vi "Midbrain.vi"() -> ()   [LabVIEW 2010]
doc: "This VI acts as the MIDbrain in the Olin Robotics Architecture. It interacts with neural clusters on both the Forebrain and Hindbrain as shown in teh respective control panel dynamic documentation diagrams."
uses:
  <vilib>/Platform/TimedLoop/XDataNode/XDataNode.xnode
  <vilib>/Platform/TimedLoop/XDataNode/timing_clust.ctl
  <vilib>/Platform/TimedLoop/XDataNode/nitl_modes.ctl
  <vilib>/Platform/TimedLoop/XDataNode/wakeup.ctl
  GlobalHowAmI.vi
  GlobalACT.vi
  GlobalWhatAroundMe.vi
  GlobalWhereAmI.vi
  <vilib>/Platform/TimedLoop/XDataNode/XDNodeRunTimeDep.lvlib
panel:
  out "Lane Follow":dbl[](array[numeric])
  out "Wall Follow":dbl[](array[numeric])
  out "AvoidWall":dbl[](array[numeric])
  out "ObsAvoid":dbl[](array[numeric])
  out "ActCommand":dbl[](array[numeric])
  out "Act Command":cluster{"Velocity":dbl, "Direction":dbl}
  out "WhereAmI? Clean":T1
  out "HowAmI? Clean":cluster{"T":dbl, "Battery":dbl, "Temp":dbl}
  out "WhatAroundMe? Clean":cluster{"T":dbl, "Range":dbl, "Bearing":dbl}[](array[cluster])
  out "Cerr":bool
  out "Limbic":bool
  out "How?":bool
  out "Act":bool
  out "What?":bool
  in  "RT-stop":bool
  out "Where?":bool
  # "must un-stop for new run"
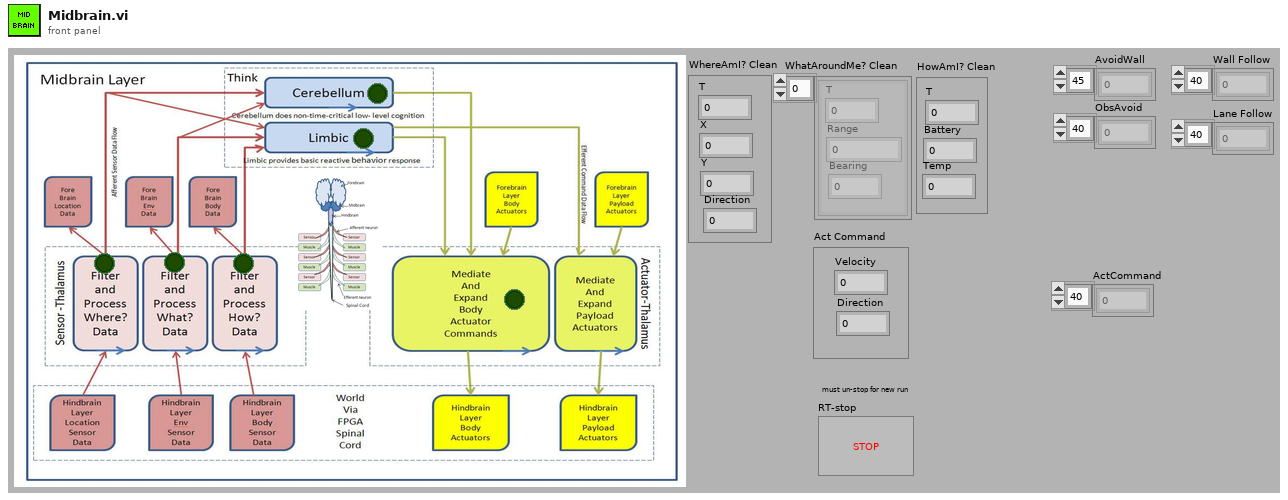
[diagram p1: front panel]
types:
  T1 = cluster{"T":dbl, "X":dbl, "Y":dbl, "Direction":dbl}
  T2 = typedef "XDNodeRunTimeDep.lvlib/timing_clust.ctl" = cluster{"Expected End [f-1]":u64, "Actual End [f-1]":u64, "Finished Late? [f-1]":bool, "Expected End [i-1]":u64, "Actual End [i-1]":u64, "Finished Late? [i-1]":bool, "Expected Start [i]":u64, "Actual Start [i]":u64, "Expected Start [f]":u64, "Actual Start [f]":u64, "Source Name":string, "Structure Name":string, "Period":i64, "Deadline":i64, "Offset":i64, "Start":i64, "Priority":i32, "Timeout":i32, "Mode":T3, "Wakeup Reason":T4, "Error":errorcluster, "Source Type":string, "Secondary Source Type":string, "Global End Time":u64, "Global Start Time":u64, "Frame Duration":u64, "Iteration Duration":u64, "Assigned CPU":i32, "I/O Scan Engine Mode":u32}
  T3 = typedef "XDNodeRunTimeDep.lvlib/nitl_modes.ctl" = enum32{"No Change", "Process missed periods, maintain original phase", "Discard missed periods, maintain original phase", "Process missed periods, ignore original phase", "Discard missed periods, ignore original phase"}
  T4 = typedef "XDNodeRunTimeDep.lvlib/wakeup.ctl" = enum32{"Normal", "Aborted", "Asynchronous wakeup", "Timing source error", "Timed loop error", "Timeout"}
  T5 = cluster{"VelCom":dbl, "BehCom":enum16{"OpenFieldTransit", "WallFollow", "LaneFollow", "ManualMode"}}
  T6 = cluster{"AvoidWall":bool, "Wander":bool, "WallFollow":bool, "LaneFollow":bool}
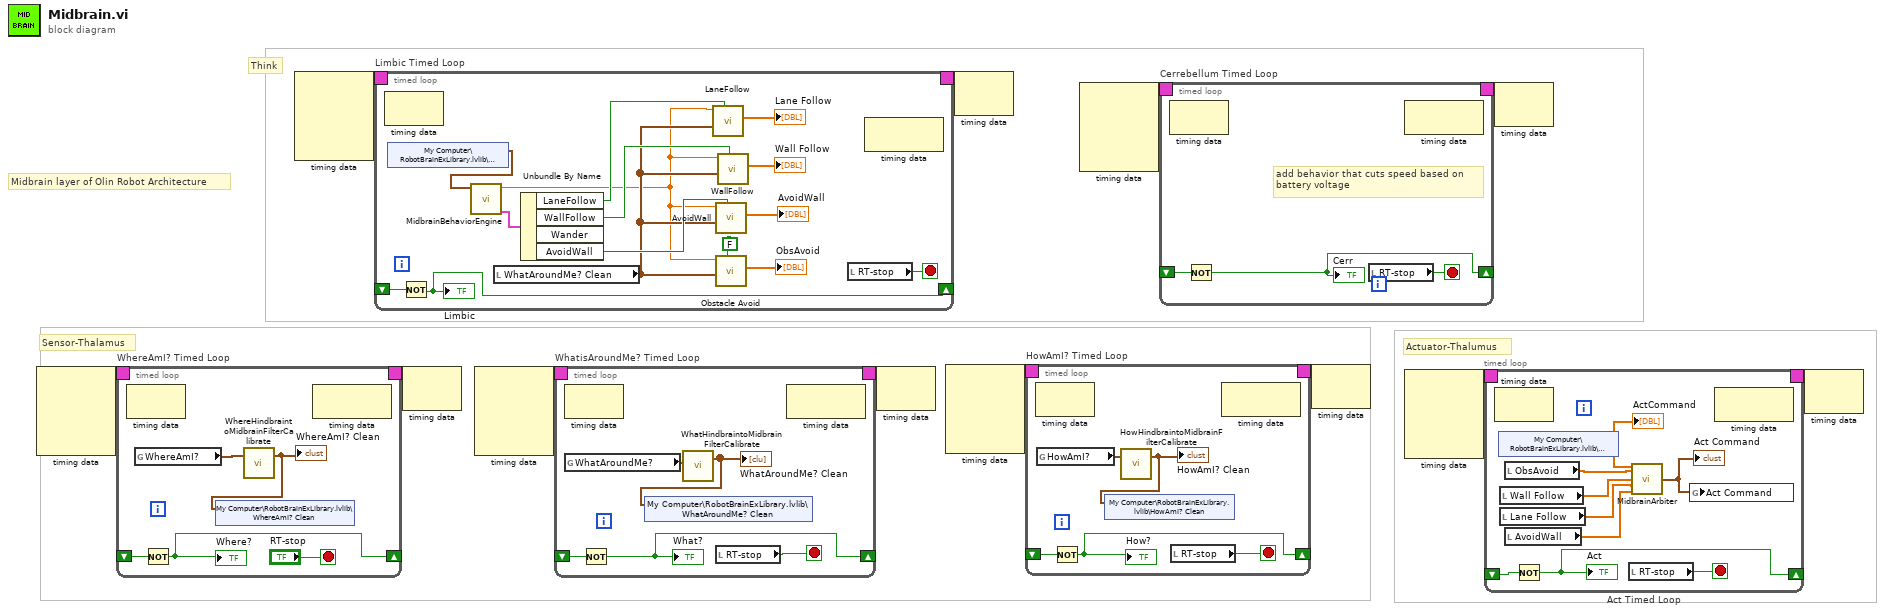
[diagram p0: block diagram]
diagram:
  # "Midbrain layer of Olin Robot Architecture"
  # "Think"
  # "Actuator-Thalumus"
  # "Sensor-Thalamus"
  n1 = node-c288 ("Input Node")() -> (w12:T2)  [unwired: 4 in]
  n2 = timed-loop "WhereAmI? Timed Loop" {
    timing: w12 -> [_]
    timing-out: [_] -> w11
    shift-right: [w16] -> _
    shift-left: _ -> [w17]
    stop <- "RT-stop" stop-if-true
    n3 = node-c288() -> ()  [unwired: 1 in, 1 out]
    n4 = global read "GlobalWhereAmI.vi" "WhereAmI?"() -> (w14:T1)
    n5 = Not(x=w17) -> (.not. x?=w16:bool)
    "Where?" <- w16
    n6 = call "WhereHindbraintoMidbrainFilterCalibrate.vi"("WhereAmI? Raw"=w14) -> ("WhereAmI? Clean"=w13:T1)  [unwired: 2 in]
    "WhereAmI? Clean" <- w13
    n7 = shared-variable "My Computer\\RobotBrainExLibrary.lvlib\\WhereAmI? Clean"(w13) -> ()  [unwired: 1 in, 1 out]
    n8 = node-c288() -> ()  [unwired: 1 in, 1 out]
  }
  n9 = node-c288 ("Input Node")() -> (w4:T2)  [unwired: 4 in]
  n10 = timed-loop "Limbic Timed Loop" {
    timing: w4 -> [_]
    timing-out: [_] -> w3
    shift-right: [w27] -> _
    shift-left: _ -> [w34]
    stop <- w33 stop-if-true
    n11 = node-c288() -> ()  [unwired: 1 in, 1 out]
    n12 = shared-variable "My Computer\\RobotBrainExLibrary.lvlib\\ForebrainCom"() -> (w31:T5)  [unwired: 1 in, 1 out]
    n13 = Not(x=w34) -> (.not. x?=w27:bool)
    "Limbic" <- w27
    n14 = call "MidbrainBehaviorEngine.vi"("ForebrainCom"=w31) -> ("BehaviorInhibit"=w26:T6, "VelCom"=w21:dbl)  [unwired: 9 in]
    n15 = local read "WhatAroundMe? Clean"() -> (w23:cluster{"T":dbl, "Range":dbl, "Bearing":dbl}[])
    n16 = Unbundle By Name(w26) -> ("LaneFollow"=w22:bool, "WallFollow"=w24:bool, "AvoidWall"=w25:bool)  [unwired: 1 out]
    n17 = call "LaneFollow.vi"("Inhibit"=w22, "WhatAroundMe? Clean"=w23, "Velocity"=w21) -> ("ActCommand"=→"Lane Follow":dbl[])  [unwired: 6 in, 2 out]
    n18 = call "AvoidWall.vi"("Inhibit"=w25, "WhatAroundMe? Clean"=w23, "Velocity"=w21) -> ("ActCommand"=→"AvoidWall":dbl[])  [unwired: 7 in, 1 out]
    n19 = call "Obstacle Avoid.vi"("Inhibit"=FALSE, "WhatAroundMe? Clean"=w23, "VelCom"=w21) -> ("ActCommand"=→"ObsAvoid":dbl[])  [unwired: 7 in, 1 out]
    n20 = call "WallFollow.vi"("Inhibit"=w24, "WhatAroundMe? Clean"=w23, "Velocity"=w21) -> ("ActCommand"=→"Wall Follow":dbl[])  [unwired: 6 in, 2 out]
    n21 = local read "RT-stop"() -> (w33:bool)
    n22 = node-c288() -> ()  [unwired: 1 in, 1 out]
  }
  n23 = node-c288(w11) -> ()  [unwired: 1 out]
  n24 = node-c288 ("Input Node")() -> (w10:T2)  [unwired: 4 in]
  n25 = timed-loop "WhatisAroundMe? Timed Loop" {
    timing: w10 -> [_]
    timing-out: [_] -> w9
    shift-right: [w40] -> _
    shift-left: _ -> [w41]
    stop <- w39 stop-if-true
    n26 = node-c288() -> ()  [unwired: 1 in, 1 out]
    n27 = global read "GlobalWhatAroundMe.vi" "WhatAroundMe?"() -> (w38:cluster{"T":dbl, "Range":dbl, "Bearing":dbl}[])
    n28 = Not(x=w41) -> (.not. x?=w40:bool)
    "What?" <- w40
    n29 = call "WhatHindbraintoMidbrainFilterCalibrate.vi"("WhatAroundMe?"=w38) -> ("WhatAroundMe? Clean"=w37:cluster{"T":dbl, "Range":dbl, "Bearing":dbl}[])  [unwired: 2 in]
    "WhatAroundMe? Clean" <- w37
    n30 = shared-variable "My Computer\\RobotBrainExLibrary.lvlib\\WhatAroundMe? Clean"(w37) -> ()  [unwired: 1 in, 1 out]
    n31 = local read "RT-stop"() -> (w39:bool)
    n32 = node-c288() -> ()  [unwired: 1 in, 1 out]
  }
  n33 = node-c288(w9) -> ()  [unwired: 1 out]
  n34 = node-c288 ("Input Node")() -> (w6:T2)  [unwired: 4 in]
  n35 = node-c288(w3) -> ()  [unwired: 1 out]
  n36 = timed-loop "HowAmI? Timed Loop" {
    timing: w6 -> [_]
    timing-out: [_] -> w5
    shift-right: [w44] -> _
    shift-left: _ -> [w48]
    stop <- w47 stop-if-true
    n37 = node-c288() -> ()  [unwired: 1 in, 1 out]
    n38 = global read "GlobalHowAmI.vi" "HowAmI?"() -> (w46:cluster{"T":dbl, "Battery":dbl, "Temp":dbl})
    n39 = Not(x=w48) -> (.not. x?=w44:bool)
    "How?" <- w44
    n40 = call "HowHindbraintoMidbrainFilterCalibrate.vi"("HowAmI?"=w46) -> ("HowAmI? Clean"=w45:cluster{"T":dbl, "Battery":dbl, "Temp":dbl})  [unwired: 2 in]
    "HowAmI? Clean" <- w45
    n41 = shared-variable "My Computer\\RobotBrainExLibrary.lvlib\\HowAmI? Clean"(w45) -> ()  [unwired: 1 in, 1 out]
    n42 = local read "RT-stop"() -> (w47:bool)
    n43 = node-c288() -> ()  [unwired: 1 in, 1 out]
  }
  n44 = node-c288 ("Input Node")() -> (w2:T2)  [unwired: 4 in]
  n45 = timed-loop "Cerrebellum Timed Loop" {
    timing: w2 -> [_]
    timing-out: [_] -> w1
    shift-right: [w52] -> _
    shift-left: _ -> [w53]
    stop <- w51 stop-if-true
    # "add behavior that cuts speed based on \nbattery voltage"
    n46 = node-c288() -> ()  [unwired: 1 in, 1 out]
    n47 = Not(x=w53) -> (.not. x?=w52:bool)
    "Cerr" <- w52
    n48 = local read "RT-stop"() -> (w51:bool)
    n49 = node-c288() -> ()  [unwired: 1 in, 1 out]
  }
  n50 = node-c288(w5) -> ()  [unwired: 1 out]
  n51 = node-c288 ("Input Node")() -> (w8:T2)  [unwired: 4 in]
  n52 = timed-loop "Act Timed Loop" {
    timing: w8 -> [_]
    timing-out: [_] -> w7
    shift-right: [w63] -> _
    shift-left: _ -> [w64]
    stop <- w62 stop-if-true
    n53 = node-c288() -> ()  [unwired: 1 in, 1 out]
    n54 = shared-variable "My Computer\\RobotBrainExLibrary.lvlib\\ActCommand"() -> (w60:dbl[])  [unwired: 1 in, 1 out]
    "ActCommand" <- w60
    n55 = local read "Wall Follow"() -> (w57:dbl[])
    n56 = local read "Lane Follow"() -> (w56:dbl[])
    n57 = local read "ObsAvoid"() -> (w59:dbl[])
    n58 = local read "AvoidWall"() -> (w58:dbl[])
    n59 = Not(x=w64) -> (.not. x?=w63:bool)
    "Act" <- w63
    n60 = local read "RT-stop"() -> (w62:bool)
    n61 = call "MidbrainArbiter.vi"("ForebrainInput"=w60, "ObstacleAvoid"=w59, "Wall Follow"=w57, "Lane Follow"=w56, "Wall Avoid"=w58) -> ("Act Command"=w61:cluster{"Velocity":dbl, "Direction":dbl})  [unwired: 10 in]
    "Act Command" <- w61
    n62 = global write "GlobalACT.vi" "Act Command"(w61) -> ()
    n63 = node-c288() -> ()  [unwired: 1 in, 1 out]
  }
  n64 = node-c288(w1) -> ()  [unwired: 1 out]
  n65 = node-c288(w7) -> ()  [unwired: 1 out]
